vi "多任务同步.vi"() -> ()   [LabVIEW 2013]
uses:
  <userlib>/ArtDAQ/_SubVI/ArtDAQ_CreateAIVoltageChan.vi
  <userlib>/ArtDAQ/_SubVI/ArtDAQ_CfgSampClkTiming.vi
  <userlib>/ArtDAQ/_SubVI/ArtDAQ_CreateAOVoltageChan.vi
  <userlib>/ArtDAQ/_SubVI/ArtDAQ_CfgDigEdgeStartTrig.vi
  <userlib>/ArtDAQ/_SubVI/ArtDAQ_Write Analog DBL 1Chan NSamp.vi
  <userlib>/ArtDAQ/_SubVI/ArtDAQ_Read Analog DBL NChan NSamp.vi
  <vilib>/Analysis/NI_AALBase.lvlib
panel:
  in  "?":enum32{"数字边沿触发"}(tab)
  in  "触发源":string="/Dev1/PFI1"
  in  "触发边沿":i32(ring)=10280 items=["上升"=10280, "下降"=10171]
  out "模拟输出":dbl[](graph)
  out "模拟输入":dbl[][](graph)
  in  "模拟输出通道":string(combo)="Dev1/ao0"
  in  "模拟输入通道":string(combo)="Dev1/ai0"
  out "ErrorOutput":errorcluster
  in  "Stop":bool
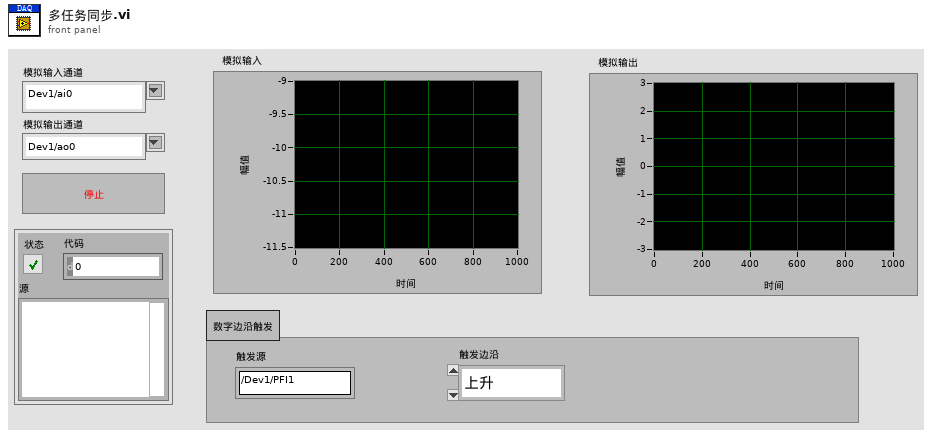
[diagram p1: front panel]
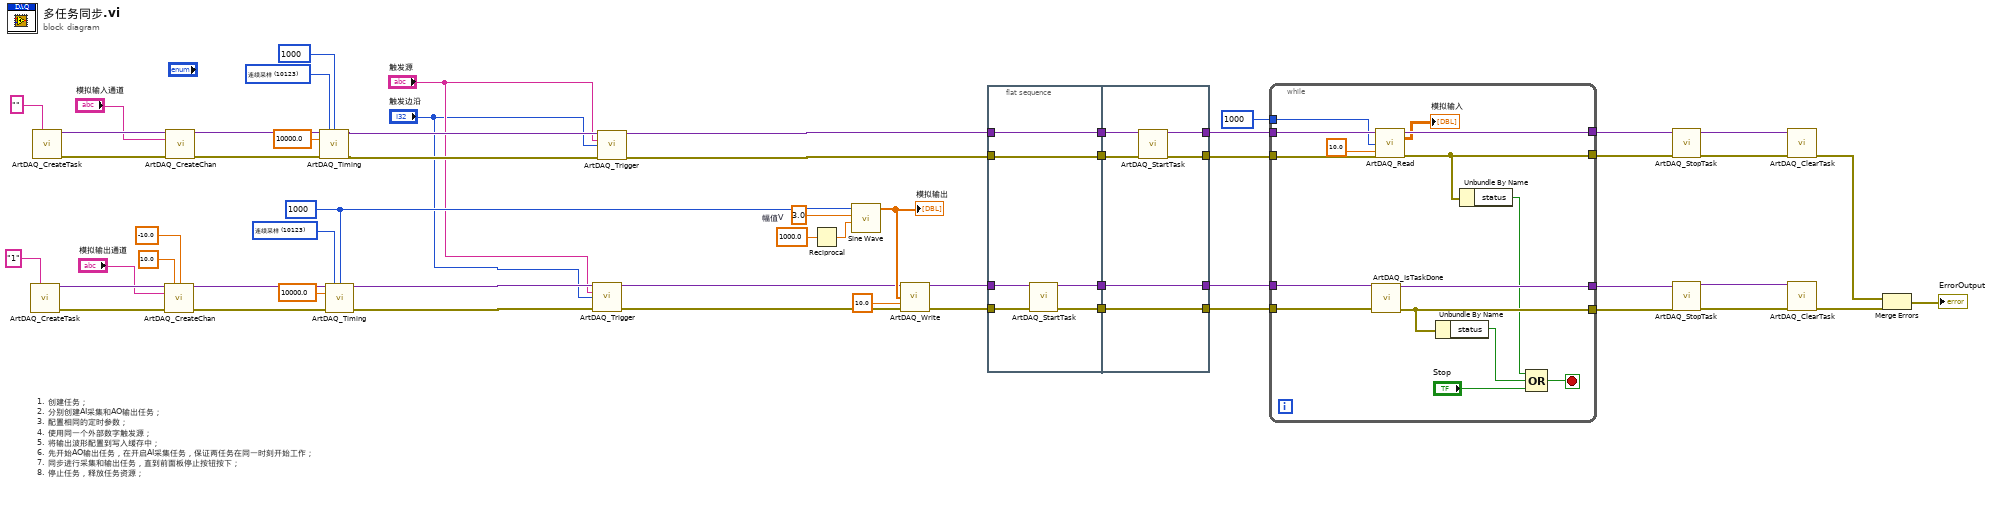
[diagram p0: block diagram]
diagram:
  w1 = 10123 items=["有限点采样"=10178, "连续采样"=10123] ("采样模式")
  w17 = 3.0  # 幅值V
  w29 = 1000 ("SamplePerChan")
  w32 = 10123 items=["有限点采样"=10178, "连续采样"=10123] ("采样模式")
  # "1. 创建任务；\n2. 分别创建AI采集和AO输出任务；\n3. 配置相同的定时参数；\n4. 使用同一个外部数字触发源；\n5. 将输出波形配置到写入缓存中；\n6. 先开始AO输出任务，在开启AI采集任务，保证两任务在同一时刻开始工作；\n7. 同步进行采集和输出任务，直到前面板停止按钮按下；\n8. 停止任务，释放任务资源；"
  n1 = call <userlib>:"ArtDAQ_CreateTask.vi"("任务名称"="1" ("TaskName")) -> ("任务句柄"=w24:variant, "错误输出"=w25:errorcluster)  [unwired: 13 in]
  n2 = call <userlib>:"ArtDAQ_CreateTask.vi"("任务名称"="" ("TaskName")) -> ("任务句柄"=w57:variant, "错误输出"=w56:errorcluster)  [unwired: 13 in]
  n3 = call-poly <userlib>:"ArtDAQ_CreateChan.vi"("任务句柄"=w24, "最大值"=10.0 ("MaxVal"), "最小值"=-10.0 ("MinVal"), "物理通道"="模拟输出通道", "错误输入"=w25) -> ("任务句柄"=w26:variant, "错误输出"=w27:errorcluster)  [unwired: 9 in]
  n4 = call-poly <userlib>:"ArtDAQ_CreateChan.vi"("任务句柄"=w57, "物理通道"="模拟输入通道", "错误输入"=w56) -> ("任务句柄"=w55:variant, "错误输出"=w54:errorcluster)  [unwired: 11 in]
  n5 = call-poly <userlib>:"ArtDAQ_Timing.vi"("任务句柄"=w55, "采样模式"=w32, "每通道采样数"=1000 ("SamplePerChan"), "采样率"=10000.0 ("Rate"), "错误输入"=w54) -> ("任务句柄"=w11:variant, "错误输出"=w10:errorcluster)  [unwired: 9 in]
  n6 = call-poly <userlib>:"ArtDAQ_Timing.vi"("任务句柄"=w26, "采样模式"=w1, "每通道采样数"=w29, "采样率"=10000.0 ("Rate"), "错误输入"=w27) -> ("任务句柄"=w7:variant, "错误输出"=w6:errorcluster)  [unwired: 9 in]
  n7 = call-poly <userlib>:"ArtDAQ_Trigger.vi"("任务句柄"=w7, "触发源"="触发源", "边沿"="触发边沿", "错误输入"=w6) -> ("任务句柄"=w4:variant, "错误输出"=w5:errorcluster)  [unwired: 10 in]
  n8 = call-poly <userlib>:"ArtDAQ_Trigger.vi"("任务句柄"=w11, "触发源"="触发源", "边沿"="触发边沿", "错误输入"=w10) -> ("任务句柄"=w9:variant, "错误输出"=w8:errorcluster)  [unwired: 10 in]
  n9 = Reciprocal(x=1000.0 ("数字")) -> (1/x=w18:dbl)
  n10 = call <vilib>:"Sine Wave.vi"("samples"=w29, "amplitude"=w17, "frequency"=w18) -> ("sine wave"=w14:dbl[])  [unwired: 2 in, 2 out]
  "模拟输出" <- w14
  n11 = call-poly <userlib>:"ArtDAQ_Write.vi"("任务句柄"=w4, "数据"=w14, "超时s"=10.0 ("Timeout"), "错误输入"=w5) -> ("任务句柄"=w40:variant, "错误输出"=w39:errorcluster)  [unwired: 9 in, 1 out]
  n12 = flat-sequence {
    tunnel: w40 -> [w63]
    tunnel: w39 -> [w62]
    tunnel: [w61] -> w46
    tunnel: [w60] -> w45
    tunnel: w9 -> [w59]
    tunnel: [w59] -> w44
    tunnel: w8 -> [w58]
    tunnel: [w58] -> w43
    tunnel: w46 -> [w65]
    tunnel: w45 -> [w64]
    tunnel: w44 -> [w69]
    tunnel: w43 -> [w68]
    tunnel: [w67] -> w38
    tunnel: [w66] -> w37
    tunnel: [w65] -> w36
    tunnel: [w64] -> w35
    frame #0 {
      n13 = call <userlib>:"ArtDAQ_StartTask.vi"("任务句柄"=w63, "错误输入"=w62) -> ("任务句柄"=w61:variant, "错误输出"=w60:errorcluster)  [unwired: 12 in]
    }
    frame #1 {
      n14 = call <userlib>:"ArtDAQ_StartTask.vi"("任务句柄"=w69, "错误输入"=w68) -> ("任务句柄"=w66:variant, "错误输出"=w67:errorcluster)  [unwired: 12 in]
    }
  }
  n15 = while {
    tunnel: w38 -> [w84]
    tunnel: [w83] -> w42
    tunnel: [w74] -> w41
    tunnel: [w82] -> w34
    tunnel: [w76] -> w33
    tunnel: w37 -> [w81]
    tunnel: w36 -> [w80]
    tunnel: w35 -> [w79]
    tunnel: 1000 ("NumSampsPerChan") -> [w70]
    stop <- w77 stop-if-true
    n16 = call <userlib>:"ArtDAQ_IsTaskDone.vi"("任务句柄"=w80, "错误输入"=w79) -> ("任务句柄"=w82:variant, "错误输出"=w76:errorcluster)  [unwired: 11 in, 1 out]
    n17 = call-poly <userlib>:"ArtDAQ_Read.vi"("任务句柄"=w81, "每通道采样数"=w70, "超时s"=10.0 ("Timeout"), "错误输入"=w84) -> ("任务句柄"=w83:variant, "数据"=→"模拟输入":dbl[][], "错误输出"=w74:errorcluster)  [unwired: 7 in, 2 out]
    n18 = Unbundle By Name(w76) -> ("status"=w75:bool)
    n19 = Unbundle By Name(w74) -> ("status"=w73:bool)
    n20 = Compound Arithmetic op=OR(w73, w75, "Stop") -> (w77:bool)
  }
  n21 = call <userlib>:"ArtDAQ_StopTask.vi"("任务句柄"=w42, "错误输入"=w41) -> ("任务句柄"=w53:variant, "错误输出"=w52:errorcluster)  [unwired: 12 in]
  n22 = call <userlib>:"ArtDAQ_StopTask.vi"("任务句柄"=w34, "错误输入"=w33) -> ("任务句柄"=w12:variant, "错误输出"=w13:errorcluster)  [unwired: 12 in]
  n23 = call <userlib>:"ArtDAQ_ClearTask.vi"("任务句柄"=w53, "错误输入"=w52) -> ("错误输出"=w50:errorcluster)  [unwired: 13 in]
  n24 = call <userlib>:"ArtDAQ_ClearTask.vi"("任务句柄"=w12, "错误输入"=w13) -> ("错误输出"=w51:errorcluster)  [unwired: 13 in]
  n25 = Merge Errors(w50, w51) -> (→"ErrorOutput":errorcluster)
